vi "polar_angle_direction.vi"(8 "error in (no error)":errorcluster, 10 "SpaceVector vector":refnum<class "SpaceVector.lvclass">, 11 "SpaceVector reference":refnum<class "SpaceVector.lvclass">) -> (0 "error out":errorcluster, 1 "r":dbl, 2 "angle":dbl, 3 "SpaceVector out":refnum<class "SpaceVector.lvclass">)   [LabVIEW 2010, in "SpaceVector.lvclass"]
uses:
  SpaceVector.lvclass
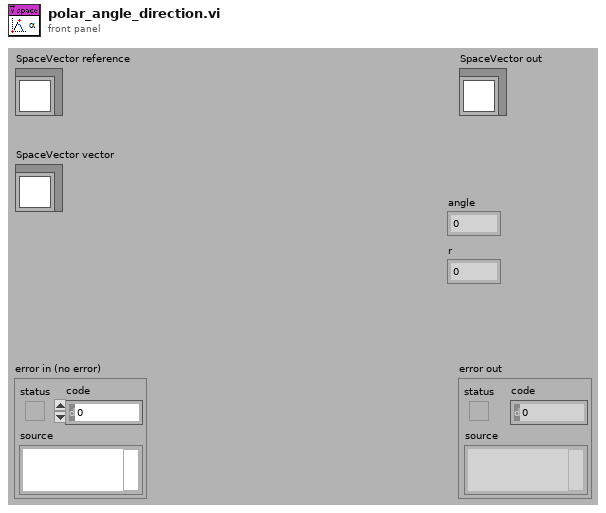
[diagram p1: front panel]
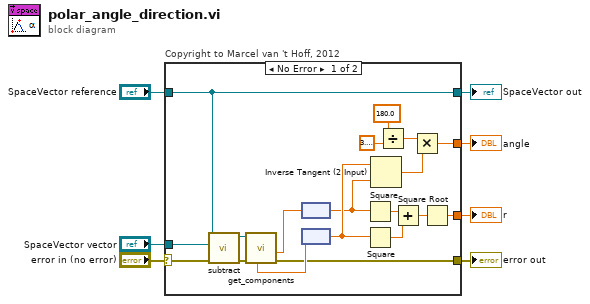
[diagram p0: block diagram]
diagram:
  n1 = case "Copyright to Marcel van 't Hoff, 2012" shown="No Error" "error in (no error)" {
    selector: "error in (no error)" -> [w9 w28]
    tunnel: [w8 w28] -> w6
    tunnel: [w11 w27] -> w4
    tunnel: "SpaceVector reference" -> [w11 w27]
    tunnel: "SpaceVector vector" -> [w12 _]
    tunnel: [w20 _] -> w2
    tunnel: [w13 _] -> w1
    frame No Error {
      n2 = call "subtract.vi"("error in (no error)"=w9, "subtrahend"=w12, "SpaceVector in"=w11) -> ("error out"=w10:errorcluster, "SpaceVector out"=w26:refnum<class "SpaceVector.lvclass">)  [unwired: 7 in]
      n3 = call "get_components.vi"("error in (no error)"=w10, "SpaceVector in"=w26) -> ("error out"=w8:errorcluster, "x"=w25:dbl[unit], "y"=w24:dbl[unit])  [unwired: 4 in, 3 out]
      n4 = node(w25) -> (w14:dbl)
      n5 = node(w24) -> (w15:dbl)
      n6 = Square(x=w14) -> (x^2=w23:dbl)
      n7 = Square(x=w15) -> (x^2=w22:dbl)
      n8 = Inverse Tangent (2 Input)(1:w14, 2:w15) -> (0:w16:dbl)
      n9 = Divide(x=180.0, y=3.141592653589793) -> (x/y=w17:dbl)
      n10 = Add(x=w23, y=w22) -> (x+y=w21:dbl)
      n11 = Multiply(x=w17, y=w16) -> (x*y=w13:dbl)
      n12 = Square Root(x=w21) -> (sqrt(x)=w20:dbl)
    }
    frame Error {
    }
  }
  "error out" <- w6
  "SpaceVector out" <- w4
  "r" <- w2
  "angle" <- w1
